vi "Set Log Path.vi"(8 "error in (no error)":errorcluster, 11 "lpszLogPath":string) -> (0 "error out":errorcluster, 2 "function return":i32, 3 "lpszLogPath out":string)   [LabVIEW 2017, in "imgAcquisition.lvlib"]
doc: "DLLFunction int __stdcall ImageCapSetLogPath(LPCTSTR lpszLogPath);"
uses:
  imgAcquisition.lvlib
  lib/ImageCaptureDLL.dll
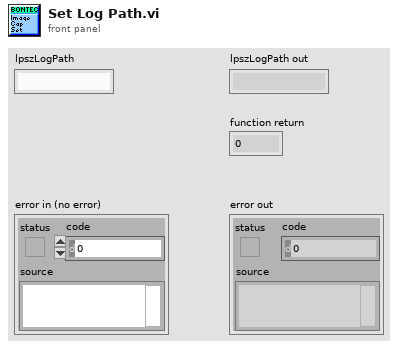
[diagram p1: front panel]
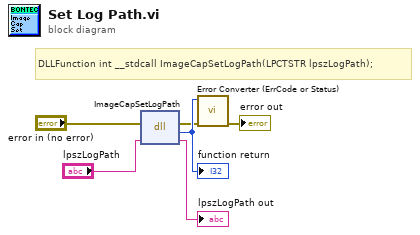
[diagram p0: block diagram]
diagram:
  # "DLLFunction int __stdcall ImageCapSetLogPath(LPCTSTR lpszLogPath);"
  n1 = dll-call lib="F:/BonTechFlatPanelLVDriver/lib/ImageCaptureDLL.*" fn="ImageCapSetLogPath"(error in="error in (no error)", "lpszLogPath"="lpszLogPath") -> (error out=w2:errorcluster, w6:i32, "lpszLogPath"=→"lpszLogPath out":string)  [unwired: 2 in, 1 out]
  "function return" <- w6
  n2 = call "Error Converter (ErrCode or Status).vi"("error in (no error)"=w2, "error code"=w6) -> ("error out"=→"error out":errorcluster)  [unwired: 9 in]
